vi "list.get_channel.vi"(8 "error in (no error)":errorcluster, 10 "index":i32, 11 "List in":refnum<class "List.lvclass">) -> (0 "error out":errorcluster, 2 "Channel":refnum<class "Channel.lvclass">, 3 "List out":refnum<class "List.lvclass">)   [LabVIEW 2020, in "List.lvclass"]
uses:
  List.lvclass
  List.lvclass/List.ctl
  Channel/Channel.lvclass
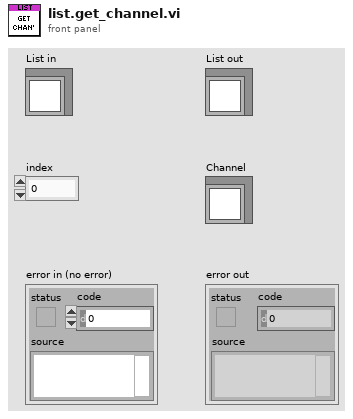
[diagram p1: front panel]
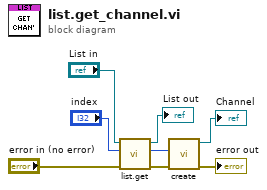
[diagram p0: block diagram]
diagram:
  n1 = call "list.get.vi"("error in"="error in (no error)", "index"="index", "List in"="List in") -> ("error out"=w7:errorcluster, "handle"=w8:i32, "List out"=→"List out":refnum<class "List.lvclass">)  [unwired: 6 in]
  n2 = call "create.vi"("error in (no error)"=w7, "handle"=w8) -> ("error out"=→"error out":errorcluster, "Channel"=→"Channel":refnum<class "Channel.lvclass">)  [unwired: 8 in]
